vi "getMaxSpeed_ShootDualTalonSRX.vi"() -> (1 "1 / Max Speed":dbl format="%.4f", 3 "Max Speed":dbl format="%.4f")   [LabVIEW 2019, in "ShootDualTalonSRX_Motor_Pair.lvlib"]
uses:
  ShootDualTalonSRX_Motor_Pair.lvlib
  globals_ShootDualTalonSRX.vi
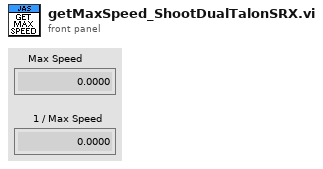
[diagram p1: front panel]
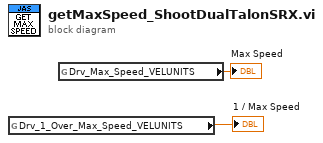
[diagram p0: block diagram]
diagram:
  n1 = global read "globals_ShootDualTalonSRX.vi" "Drv_1_Over_Max_Speed_VELUNITS"() -> (→"1 / Max Speed":dbl)
  n2 = global read "globals_ShootDualTalonSRX.vi" "Drv_Max_Speed_VELUNITS"() -> (→"Max Speed":dbl)
